vi "get mode, position, limits and name.vi"(8 "error in (no error)":errorcluster, 11 "Status":T1) -> (0 "error out":errorcluster)   [LabVIEW 2021]
uses:
  ctl/Servo over status.ctl
  ctl/Servo status variable.ctl
  ctl/Servo status constants.ctl
  <vilib>/addons/eal4LabVIEW/eal4LabVIEW.lvlib
panel:
  out "Status out":T1
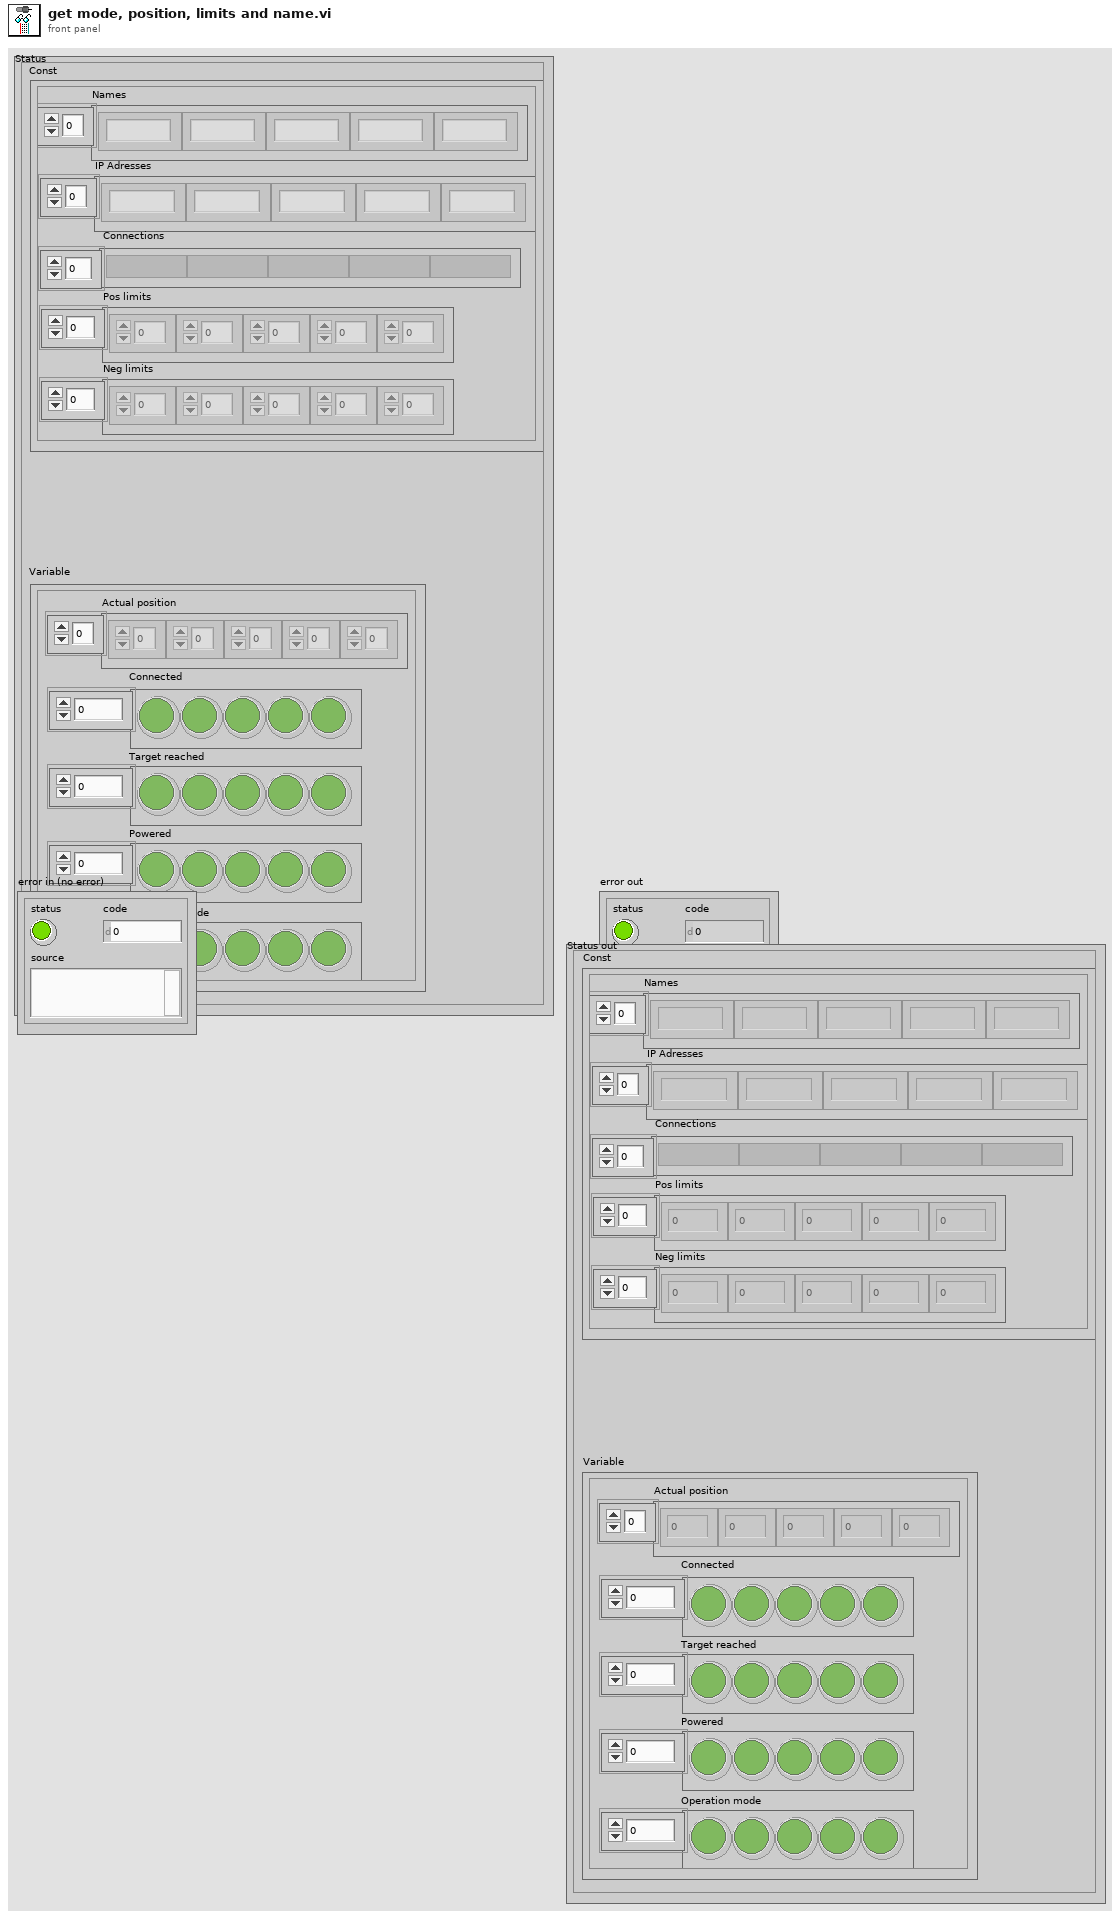
[diagram p1: front panel]
types:
  T1 = typedef "Servo over status.ctl" = cluster{"Variable":T2, "Const":T3}
  T2 = typedef "Servo status variable.ctl" = cluster{"Connected":bool[], "Target reached":bool[], "Powered":bool[], "Actual position":dbl[], "Operation mode":bool[]}
  T3 = typedef "Servo status constants.ctl" = cluster{"IP Adresses":string[], "Names":string[], "Connections":variant[], "Pos limits":dbl[], "Neg limits":dbl[]}
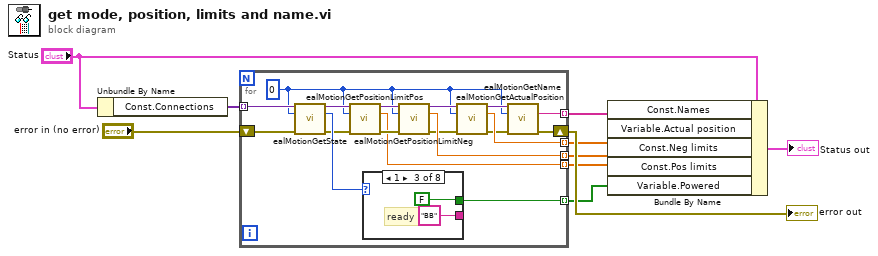
[diagram p0: block diagram]
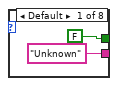
[diagram p2: hidden frame]
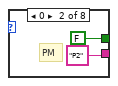
[diagram p3: hidden frame]
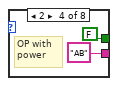
[diagram p4: hidden frame]
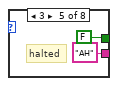
[diagram p5: hidden frame]
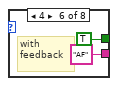
[diagram p6: hidden frame]
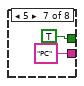
[diagram p7: hidden frame]
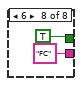
[diagram p8: hidden frame]
diagram:
  n1 = Unbundle By Name("Status") -> ("Const.Connections"=w10:variant[])
  n2 = for {
    shift-right: [w28] -> w8
    shift-left: "error in (no error)" -> [w23]
    tunnel: [w27] -> w6 mode=indexing
    tunnel: [w25] -> w3 mode=indexing
    tunnel: w10 -> [w24] mode=indexing
    tunnel: [w17] -> w5 mode=indexing
    tunnel: [w16] -> w4 mode=indexing
    tunnel: [w14] -> w2 mode=indexing
    w13 = 0 ("slave index")
    n3 = call <vilib>:"ealMotionGetState.vi"("connection in"=w24, "slave index"=w13, "error in (no error)"=w23) -> ("connection out"=w22:variant, "get state"=w26:i32, "error out"=w19:errorcluster)  [unwired: 10 in]
    n4 = call <vilib>:"ealMotionGetPositionLimitPos.vi"("connection in"=w22, "slave index"=w13, "error in (no error)"=w19) -> ("connection out"=w21:variant, "positive position limit"=w17:dbl, "error out"=w18:errorcluster)  [unwired: 10 in]
    n5 = case shown="1" w26 {
      tunnel: ["Unknown" "P2" "BB" "AB" "AH" "AF" "PC" "FC"] -> _
      tunnel: [FALSE FALSE FALSE FALSE FALSE TRUE TRUE TRUE] -> w25
      frame Default {
      }
      frame 0 {
        # "PM"
      }
      frame 1 {
        # "ready"
      }
      frame 2 {
        # "OP with\npower"
      }
      frame 3 {
        # "halted"
      }
      frame 4 {
        # "with\nfeedback"
      }
      frame 5 {
      }
      frame 6 {
      }
    }
    n6 = call <vilib>:"ealMotionGetPositionLimitNeg.vi"("connection in"=w21, "slave index"=w13, "error in (no error)"=w18) -> ("connection out"=w20:variant, "negative position limit"=w16:dbl, "error out"=w11:errorcluster)  [unwired: 10 in]
    n7 = call <vilib>:"ealMotionGetActualPosition.vi"("connection in"=w20, "slave index"=w13, "error in (no error)"=w11) -> ("connection out"=w15:variant, "getActualPosition"=w14:dbl, "error out"=w12:errorcluster)  [unwired: 10 in]
    n8 = call <vilib>:"ealMotionGetName.vi"("connection in"=w15, "slave index"=w13, "error in (no error)"=w12) -> ("name"=w27:string, "error out"=w28:errorcluster)  [unwired: 10 in, 1 out]
  }
  "error out" <- w8
  n9 = Bundle By Name(cluster="Status", "Const.Names"=w6, "Variable.Actual position"=w2, "Const.Neg limits"=w4, "Const.Pos limits"=w5, "Variable.Powered"=w3) -> (→"Status out":T1)
